vi "纳清蓝绿藻_所有参数读取.vi"(8 "error in (no error)":errorcluster caption="错误输入（无错误）", 11 "MB session in":refnum<class "MB_Master.lvclass">) -> (0 "error out":errorcluster caption="错误输出", 2 "输出值":T1 {"波特率" items=["4800", "9600", "19200", "38400", "57600", "115200"]}, 3 "MB session out":refnum<class "MB_Master.lvclass">)   [LabVIEW 2016, in "斯坦道多参数.lvlib"]
uses:
  <vilib>/Plasmionique/MB Master/MB_Master/MB_Master.lvclass
  <vilib>/Plasmionique/MB Master/MB Master.lvlib
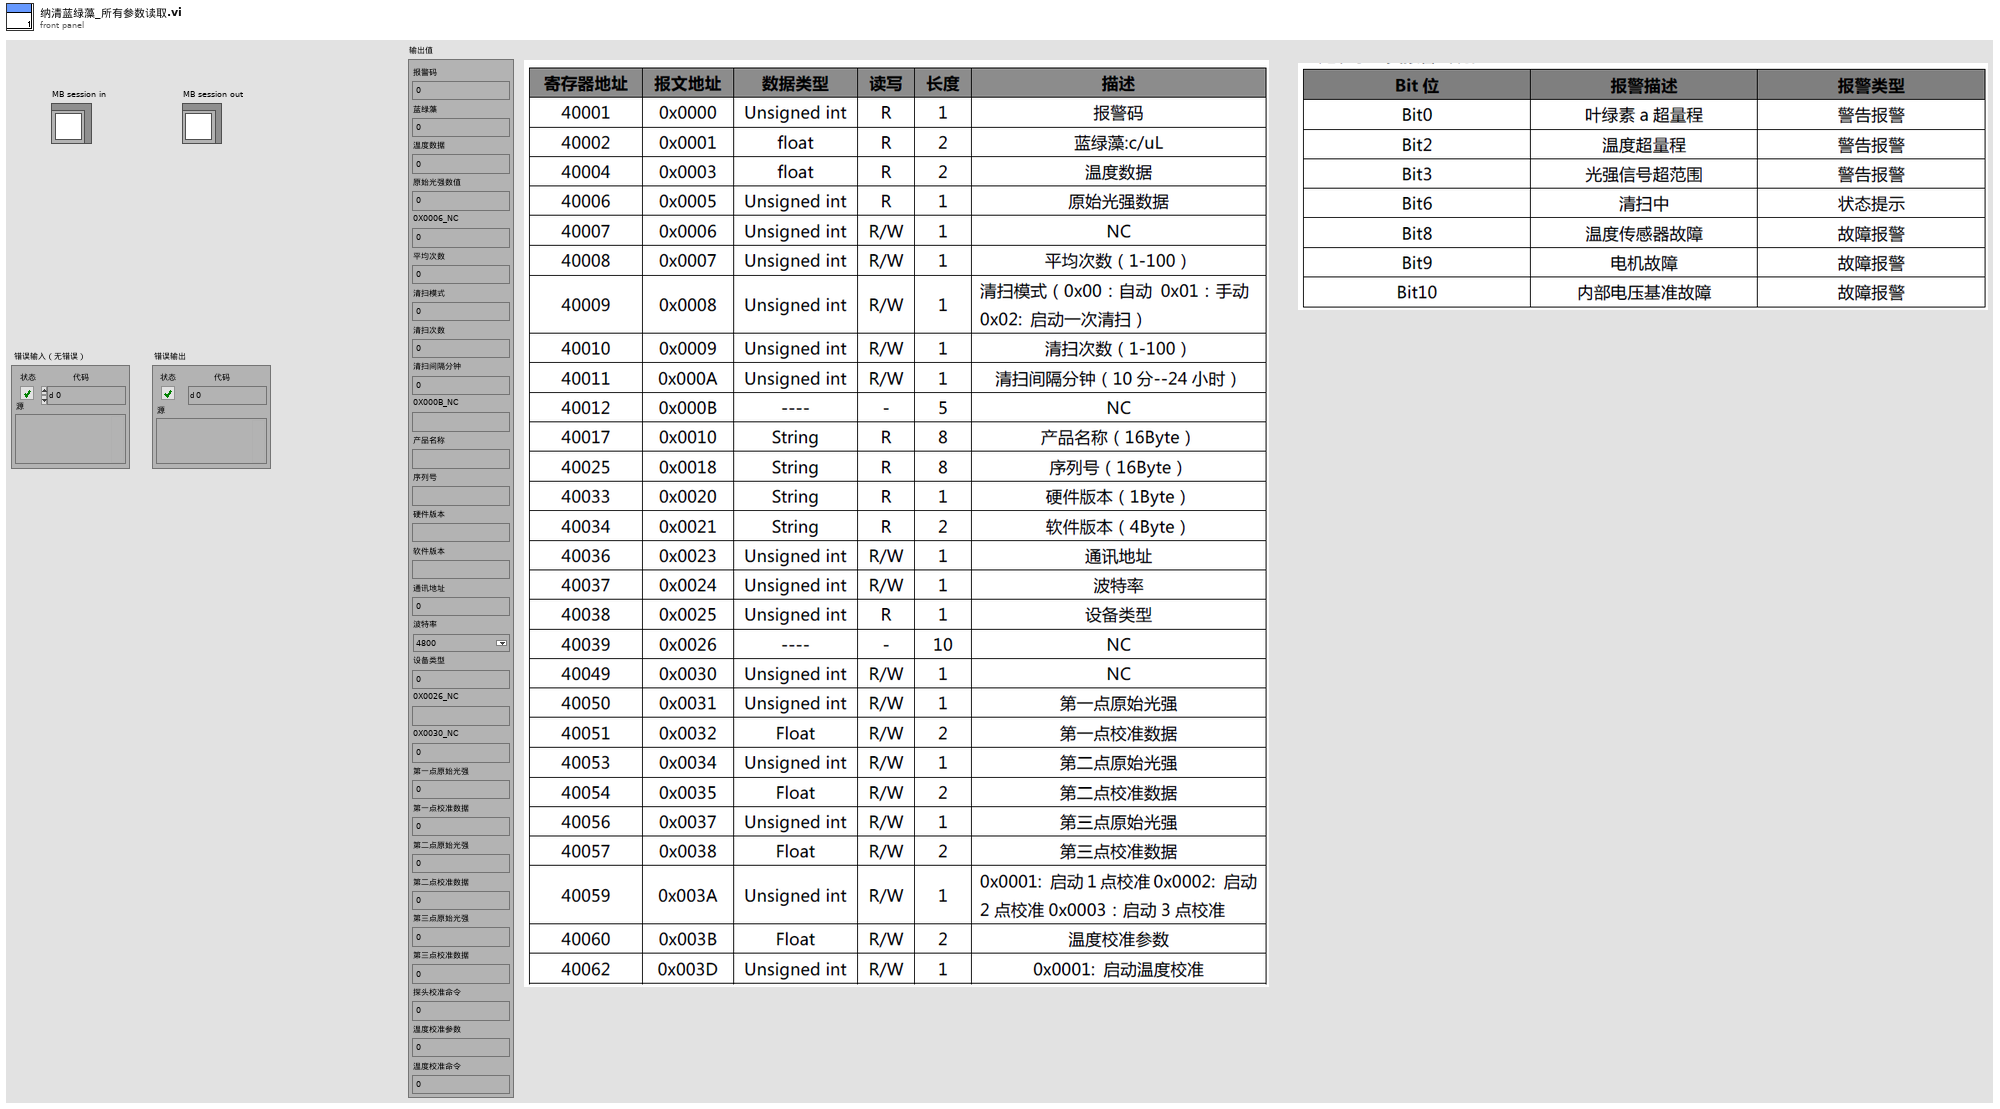
[diagram p1: front panel]
types:
  T1 = cluster{"报警码":u16, "蓝绿藻":sgl, "温度数据":sgl, "原始光强数值":u16, "0X0006_NC":u16, "平均次数":u16, "清扫模式":u16, "清扫次数":u16, "清扫间隔分钟":u16, "0X000B_NC":string, "产品名称":string, "序列号":string, "硬件版本":string, "软件版本":string, "通讯地址":u16, "波特率":u16, "设备类型":u16, "0X0026_NC":string, "0X0030_NC":u16, "第一点原始光强":u16, "第一点校准数据":sgl, "第二点原始光强":u16, "第二点校准数据":sgl, "第三点原始光强":u16, "第三点校准数据":sgl, "探头校准命令":u16, "温度校准参数":sgl, "温度校准命令":u16}
  T2 = cluster{u16, "数值":sgl, "数值":sgl, u16, u16, u16, u16, u16, u16, "类型":string, "类型":string, "类型":string, "类型":string, "类型":string, u16, u16, u16, "类型":string, u16, u16, "数值":sgl, u16, "数值":sgl, u16, "数值":sgl, u16, "数值":sgl, u16}
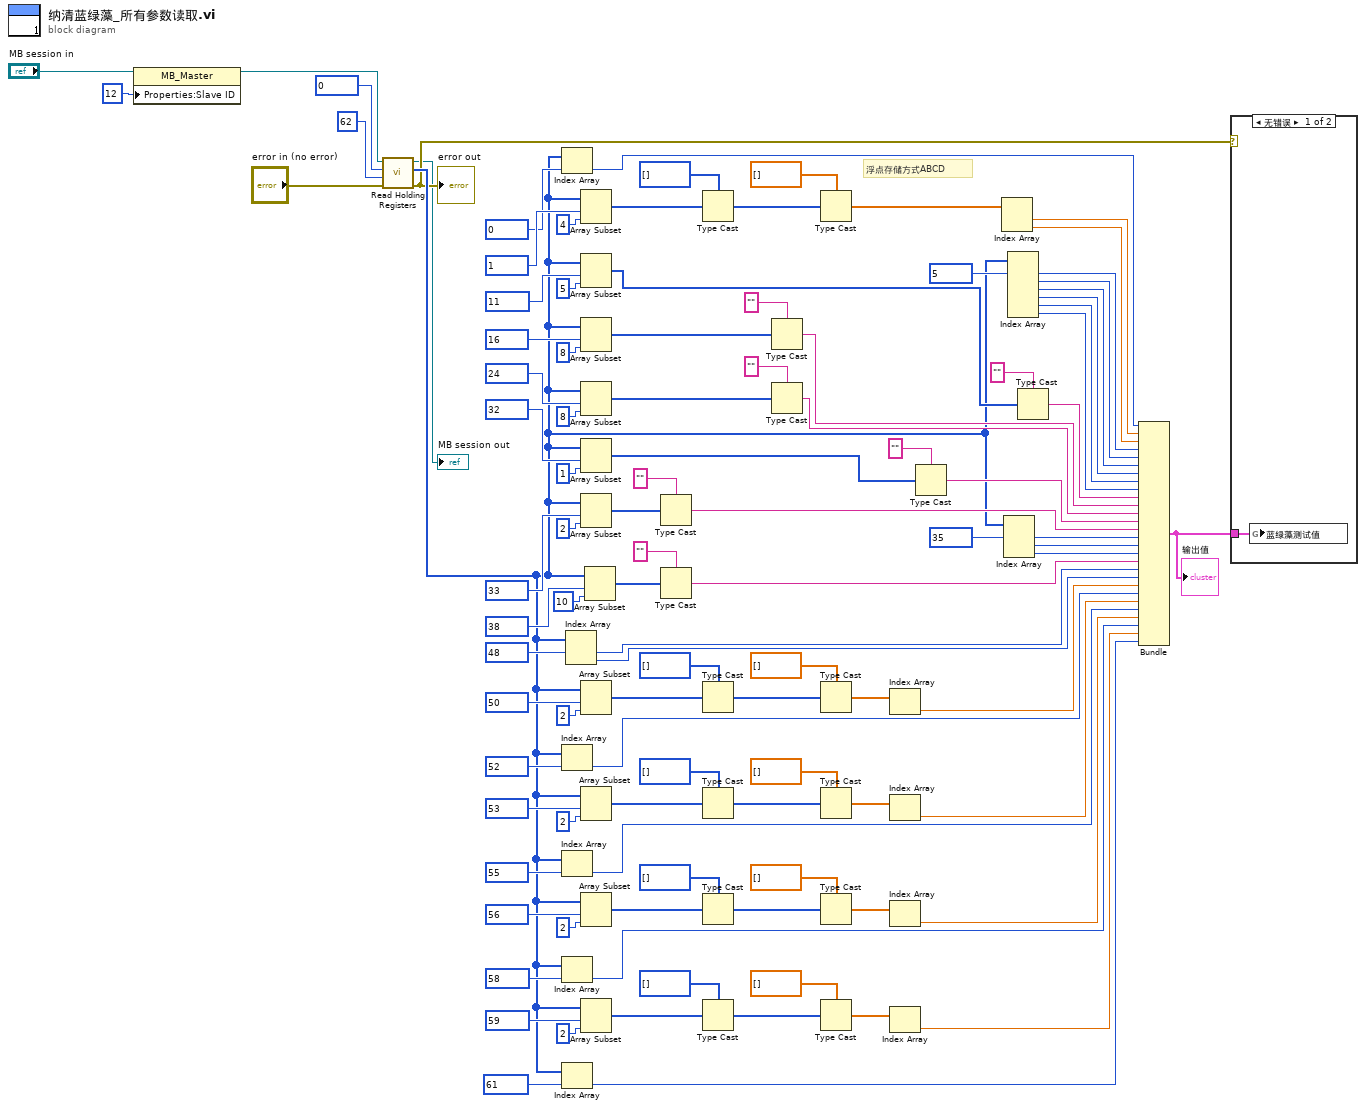
[diagram p0: block diagram]
diagram:
  # "浮点存储方式ABCD"
  n1 = property class="MB_Master"(reference="MB session in", "Properties:Slave ID"=u8 12 ("Slave ID")) -> (reference out=w95:refnum<class "MB_Master.lvclass">)  [unwired: 1 in, 1 out]
  n2 = call <vilib>:"Read Holding Registers.vi"("error in (no error)"="error in (no error)", "quantity"=u16 62, "starting address"=u16 0, "MB session in"=w95) -> ("error out"=w5:errorcluster, "Registers"=w7:u16[], "MB session out"=→"MB session out":refnum<class "MB_Master.lvclass">)  [unwired: 5 in]
  "error out" <- w5
  n3 = Index Array(array=w7, index=u16 0 ("starting address")) -> (element=w103:u16)
  n4 = Index Array(array=w7, index=u16 52 ("starting address")) -> (element=w30:u16)
  n5 = Index Array(array=w7, index=u16 55 ("starting address")) -> (element=w20:u16)
  n6 = Index Array(array=w7, index=u16 58 ("starting address")) -> (element=w10:u16)
  n7 = Index Array(array=w7, index=u16 61 ("starting address")) -> (element=w6:u16)
  n8 = Index Array(array=w7, index #1=u16 48 ("starting address")) -> (element #1=w48:u16, element #2=w47:u16)  [unwired: 1 in]
  n9 = Array Subset(array=w7, index=u16 1 ("starting address"), length=4 ("长度")) -> (w99:u16[])
  n10 = Array Subset(array=w7, index=u16 11 ("starting address"), length=5 ("长度")) -> (w81:u16[])
  n11 = Array Subset(array=w7, index=u16 16 ("starting address"), length=8 ("长度")) -> (w77:u16[])
  n12 = Array Subset(array=w7, index=u16 24 ("starting address"), length=8 ("长度")) -> (w71:u16[])
  n13 = Array Subset(array=w7, index=u16 32 ("starting address"), length=1 ("长度")) -> (w67:u16[])
  n14 = Array Subset(array=w7, index=u16 33 ("starting address"), length=2 ("长度")) -> (w61:u16[])
  n15 = Array Subset(array=w7, index=u16 50 ("starting address"), length=2 ("长度")) -> (w45:u16[])
  n16 = Array Subset(array=w7, index=u16 53 ("starting address"), length=2 ("长度")) -> (w33:u16[])
  n17 = Array Subset(array=w7, index=u16 56 ("starting address"), length=2 ("长度")) -> (w26:u16[])
  n18 = Array Subset(array=w7, index=u16 59 ("starting address"), length=2 ("长度")) -> (w13:u16[])
  n19 = Array Subset(array=w7, index=u16 38 ("starting address"), length=10 ("长度")) -> (w51:u16[])
  n20 = Type Cast(type="" ("类型"), x=w61) -> (*(type *) &x=w59:string)
  n21 = Type Cast(type="" ("类型"), x=w51) -> (*(type *) &x=w50:string)
  n22 = Type Cast(type=u32[] [] ("数组 2"), x=w99) -> (*(type *) &x=w4:u32[])
  n23 = Type Cast(type=u32[] [] ("数组 2"), x=w45) -> (*(type *) &x=w43:u32[])
  n24 = Type Cast(type=u32[] [] ("数组 2"), x=w33) -> (*(type *) &x=w35:u32[])
  n25 = Type Cast(type=u32[] [] ("数组 2"), x=w26) -> (*(type *) &x=w24:u32[])
  n26 = Type Cast(type=u32[] [] ("数组 2"), x=w13) -> (*(type *) &x=w15:u32[])
  n27 = Type Cast(type="" ("类型"), x=w77) -> (*(type *) &x=w74:string)
  n28 = Type Cast(type="" ("类型"), x=w71) -> (*(type *) &x=w69:string)
  n29 = Type Cast(type=sgl[] [] ("数组 2"), x=w4) -> (*(type *) &x=w98:sgl[])
  n30 = Type Cast(type=sgl[] [] ("数组 2"), x=w43) -> (*(type *) &x=w40:sgl[])
  n31 = Type Cast(type=sgl[] [] ("数组 2"), x=w35) -> (*(type *) &x=w38:sgl[])
  n32 = Type Cast(type=sgl[] [] ("数组 2"), x=w24) -> (*(type *) &x=w21:sgl[])
  n33 = Type Cast(type=sgl[] [] ("数组 2"), x=w15) -> (*(type *) &x=w18:sgl[])
  n34 = Index Array(array=w40) -> (element=w39:sgl)  [unwired: 1 in]
  n35 = Index Array(array=w38) -> (element=w29:sgl)  [unwired: 1 in]
  n36 = Index Array(array=w21) -> (element=w19:sgl)  [unwired: 1 in]
  n37 = Index Array(array=w18) -> (element=w9:sgl)  [unwired: 1 in]
  n38 = Type Cast(type="" ("类型"), x=w67) -> (*(type *) &x=w64:string)
  n39 = Index Array(array=w98) -> (element #1=w93:sgl, element #2=w92:sgl)  [unwired: 2 in]
  n40 = Index Array(array=w7, index #1=u16 35 ("starting address")) -> (element #1=w57:u16, element #2=w56:u16, element #3=w55:u16)  [unwired: 2 in]
  n41 = Index Array(array=w7, index #1=u16 5 ("starting address")) -> (element #1=w89:u16, element #2=w88:u16, element #3=w87:u16, element #4=w86:u16, element #5=w85:u16, element #6=w84:u16)  [unwired: 5 in]
  n42 = Type Cast(type="" ("类型"), x=w81) -> (*(type *) &x=w79:string)
  n43 = Bundle(w103, "数值"=w93, "数值"=w92, w89, w88, w87, w86, w85, w84, "类型"=w79, "类型"=w74, "类型"=w69, "类型"=w64, "类型"=w59, w57, w56, w55, "类型"=w50, w48, w47, "数值"=w39, w30, "数值"=w29, w20, "数值"=w19, w10, "数值"=w9, w6) -> (w1:T2)  [unwired: 1 in]
  "输出值" <- w1
  n44 = case shown="无错误" w5 {
    tunnel: w1 -> [w106 _]
    frame No Error {
      n45 = global write "纳清过程全局变量.vi" "蓝绿藻测试值"(w106) -> ()
    }
    frame Error {
    }
  }
